vi "Countdown.vi"(10 "Delay before logging":i32, 11 "Digital in":refnum<vi>) -> ()   [LabVIEW 2017, in "LeapMotion.lvlib"]
uses:
  LeapMotion.lvlib
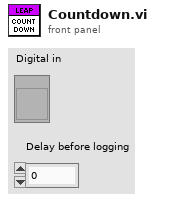
[diagram p1: front panel]
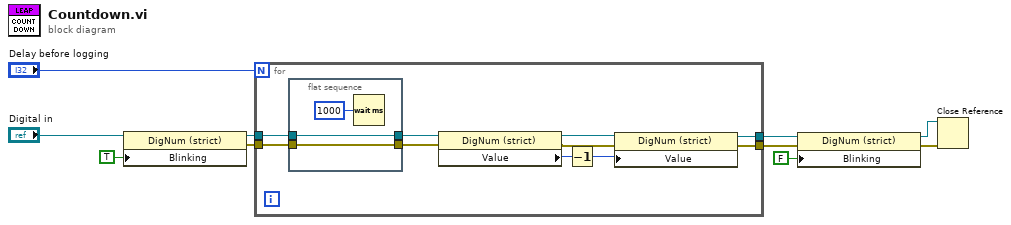
[diagram p0: block diagram]
diagram:
  n1 = property class="DigNum (strict)"(reference="Digital in", "Blinking"=TRUE) -> (reference out=w3:refnum<vi>, error out=w4:errorcluster)  [unwired: 1 in]
  n2 = for {
    N: "Delay before logging" -> [_]
    tunnel: [w16] -> w6
    tunnel: [w15] -> w7
    tunnel: w3 -> [w13]
    tunnel: w4 -> [w12]
    n3 = flat-sequence {
      tunnel: [w22] -> w14
      tunnel: w13 -> [w22]
      tunnel: w12 -> [w21]
      tunnel: [w21] -> w11
      frame #0 {
        n4 = Wait (ms)(milliseconds to wait=u32 1000) -> ()  [unwired: 1 out]
      }
    }
    n5 = property class="DigNum (strict)"(reference=w14, error in=w11) -> (reference out=w18:refnum<vi>, error out=w17:errorcluster, "Value"=w19:i32)
    n6 = Decrement(x=w19) -> (x-1=w20:i32)
    n7 = property class="DigNum (strict)"(reference=w18, error in=w17, "Value"=w20) -> (reference out=w16:refnum<vi>, error out=w15:errorcluster)
  }
  n8 = property class="DigNum (strict)"(reference=w6, error in=w7, "Blinking"=FALSE) -> (reference out=w10:refnum<vi>, error out=w9:errorcluster)
  n9 = Close Reference(reference=w10, error in (no error)=w9) -> ()  [unwired: 1 out]
